vi "ASYNC_Adam_client-cluster.vi"(1 "name-ValueArray":cluster{"String":string, "Numeric":dbl}[](array[cluster]), 4 "prefixString":string) -> (6 "Scan Comments":string[](array[string]))   [LabVIEW 2021]
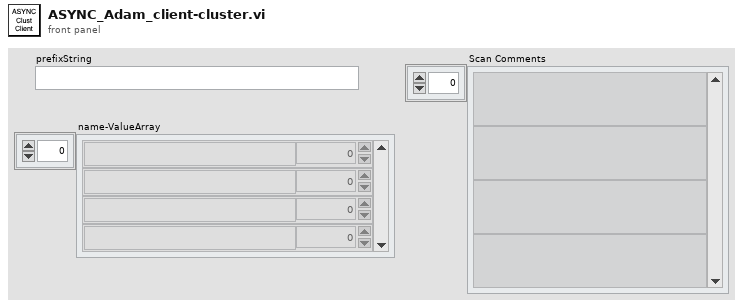
[diagram p1: front panel]
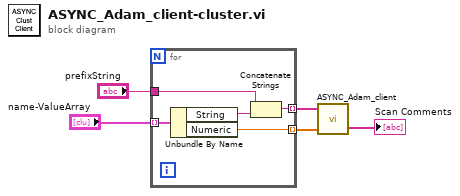
[diagram p0: block diagram]
diagram:
  n1 = for {
    tunnel: "name-ValueArray" -> [w10] mode=indexing
    tunnel: "prefixString" -> [w8]
    tunnel: [w7] -> w2 mode=indexing
    tunnel: [w6] -> w1 mode=indexing
    n2 = Unbundle By Name(w10) -> ("String"=w9:string, "Numeric"=w6:dbl)
    n3 = Concatenate Strings(w8, w9) -> (w7:string)
  }
  n4 = call "ASYNC_Adam_client.vi"("Values"=w1, "Channel Names"=w2) -> ("Scan Comments"=→"Scan Comments":string[])  [unwired: 1 in, 1 out]
